vi "Set Device Adress.vi"(4 "error in (no error)":errorcluster, 6 "Adress Number (1)":i32=1 min=1 max=30, 7 "VISA resource name":refnum<visa-resource-name>) -> (0 "error out":errorcluster, 3 "VISA resource name out":refnum<visa-resource-name>)   [LabVIEW 2012, in "Newport ESP301.lvlib"]
doc: "This command is used to set and report the device (i.e., ESP controller) address for use with IEEE-488 or USB communications (if equipped).\nThe address change takes affect immediately after the command is processed.\nNote:\nUse the \"Save Settings To Non-Volatile Memory.vi\" to save new address setting to non-volatile memory."
uses:
  Newport ESP301.lvlib
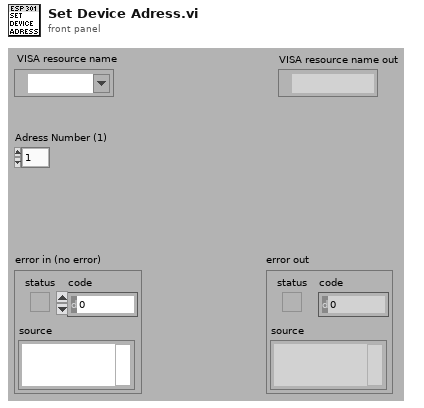
[diagram p1: front panel]
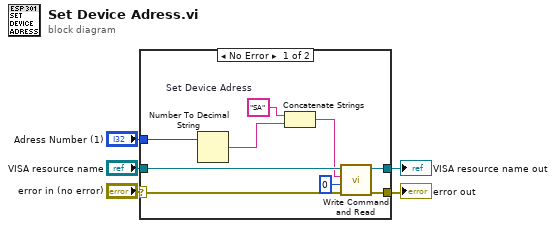
[diagram p0: block diagram]
diagram:
  n1 = case shown="No Error" "error in (no error)" {
    selector: "error in (no error)" -> [w11 w16]
    tunnel: [w13 w16] -> w5
    tunnel: "VISA resource name" -> [w14 w15]
    tunnel: [w12 w15] -> w4
    tunnel: "Adress Number (1)" -> [w8 _]
    frame No Error {
      w10 = "SA"  # Set Device Adress
      n2 = Number To Decimal String(number=w8) -> (decimal integer string=w6:string)  [unwired: 1 in]
      n3 = Concatenate Strings(w10, w6) -> (w9:string)
      n4 = call "Write Command and Read.vi"("error in (no error)"=w11, "Bytes to read (100)"=u32 0, "Command"=w9, "VISA resource name"=w14) -> ("error out"=w13:errorcluster, "VISA resource name out"=w12:refnum<visa-resource-name>)  [unwired: 3 in, 1 out]
    }
    frame Error {
    }
  }
  "error out" <- w5
  "VISA resource name out" <- w4
